vi "Engine Out - Faults - Turbo Outlet Exhaust Pressure.vi"(11 "Turbo Outlet Exhaust Pressure [kPa]":sgl) -> ()   [LabVIEW 2015, in "ECS-RT.lvlib"]
uses:
  ECS-RT.lvlib
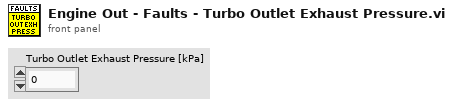
[diagram p1: front panel]
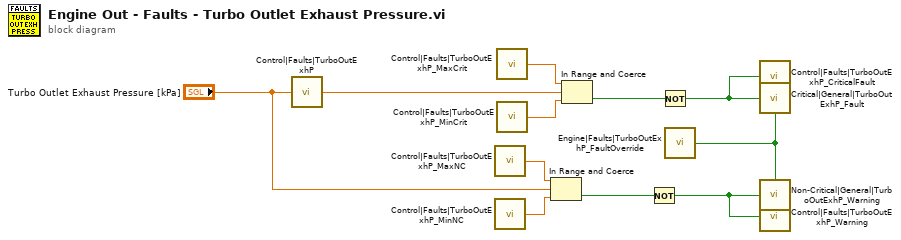
[diagram p0: block diagram]
diagram:
  n1 = call "Control|Faults|TurboOutExhP"("Value"="Turbo Outlet Exhaust Pressure [kPa]") -> ()
  n2 = call "Control|Faults|TurboOutExhP_MaxNC"() -> ("Value"=w9:sgl)
  n3 = call "Control|Faults|TurboOutExhP_MinNC"() -> ("Value"=w8:sgl)
  n4 = call "Control|Faults|TurboOutExhP_MaxCrit"() -> ("Value"=w5:sgl)
  n5 = call "Control|Faults|TurboOutExhP_MinCrit"() -> ("Value"=w4:sgl)
  n6 = In Range and Coerce(upper limit=w9, x="Turbo Outlet Exhaust Pressure [kPa]", lower limit=w8) -> (In Range?=w7:bool)  [unwired: 1 out]
  n7 = In Range and Coerce(upper limit=w5, x="Turbo Outlet Exhaust Pressure [kPa]", lower limit=w4) -> (In Range?=w3:bool)  [unwired: 1 out]
  n8 = Not(x=w7) -> (.not. x?=w10:bool)
  n9 = Not(x=w3) -> (.not. x?=w6:bool)
  n10 = call "Engine|Faults|TurboOutExhP_FaultOverride"() -> ("Value"=w1:bool)
  n11 = call "Control|Faults|TurboOutExhP_CriticalFault"("Value"=w6) -> ()
  n12 = call "Critical|General|TurboOutExhP_Fault"("Fault"=w6, "Override (F)"=w1) -> ()  [unwired: 1 in]
  n13 = call "Non-Critical|General|TurboOutExhP_Warning"("Fault"=w10, "Override (F)"=w1) -> ()  [unwired: 1 in]
  n14 = call "Control|Faults|TurboOutExhP_Warning"("Value"=w10) -> ()
